vi "XIPIN_RXAUI_4_3.vi"   [LabVIEW 2017]
doc: "The Xilinx Reduced Pin 10 Gigabit Attachment Unit Interface (RXAUI) LogiCORE provides a 2-lane high speed serial interface, providing up to 10 Gigabits per second (Gbps) total throughput. Operating at an internal clock speed of 156.25 MHz, the core includes the Dune Networks RXAUI implementation, the XGMII Extender Sublayers (DTE and PHY XGXS), and the 10GBASE-X sublayer, as described in clauses 47 and 48 of IEEE 802.3-2008. The core supports an optional serial MDIO management interface for accessing the IEEE 802.3-2008 clause 45 management registers. The MDIO interface may be omitted to save slice logic, in which case a simplified management interface is provided via bit vectors. The core is designed to seamlessly interface with the 10 Gigabit Ethernet Media Access Controller (XGMAC) LogiCORE via the XGMII.\n------------------------------------\n<b>Need License</b> : No"
uses:
  <vilib>/rvi/XilinxIP/XIPIN_XNode/niFpgaXIPIN.xnode
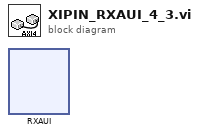
[diagram p0: block diagram]
diagram:
  n1 = xnode ("RXAUI")() -> ()
